vi "AOL Properties parser.vi"(0 "AOL Properties":T4={"AOD 1 thickness (mm)"=118.0, "AOD 2 thickness (mm)"=115.0, "AOD 3 thickness (mm)"=110.0, "AOD 4 thickness (mm)"=135.0, "AOD 1-2 separation (mm)"=135.0, "AOD 2-3 separation (mm)"=135.0, "AOD 3-4 separation (mm)"=15.0, "AOL aperture (mm)"=15.0, "AOL centre wavelength (nm)"=15.0, "AOL centre frequency (MHz)"=15.0, "skewZX"=15.0, "skewZY"=15.0, "magZX"=50.0, "magZY"=50.0, "Diffraction mode"=50.0, "Crystal length (mm)"=15.0, "Acoustic velocity (m/s)"=1.0, "Pair deflection ratio"=1.0, "AOD fill time (us)"=1.0}) -> (14 "Keys setup.DBL":T2=[{"key"="Control FPGA.Clock Freq (MHz)", "Save?"=TRUE, "Default"=240.0}, {"key"="DAQ FPGA.Clock Freq (MHz)", "Save?"=TRUE, "Default"=240.0}], 15 "Values.DBL":dbl[](array[numeric]), 16 "Keys setup.String":T3=[{"key"="Control FPGA.MAC address", "Save?"=TRUE, "Default"="AABBCCDDEEFF"}, {"key"="DAQ FPGA.Target", "Save?"=TRUE, "Default"="RIO0"}, {"key"="XY Stage.COM port", "Save?"=TRUE, "Default"="COM7"}, {"key"="DAQmx Chan.Pockels Control", "Save?"=TRUE, "Default"=""}, {"key"="DAQmx Chan.Hard Shutter", "Save?"=TRUE, "Default"=""}, {"key"="DAQmx Chan.PMT 1", "Save?"=TRUE, "Default"=""}, {"key"="DAQmx Chan.PMT 2", "Save?"=TRUE, "Default"=""}, {"key"="DAQmx Chan.Encoder Trigger", "Save?"=TRUE, "Default"=""}, {"key"="DAQmx Chan.Optional Trigger 1", "Save?"=TRUE, "Default"=""}, {"key"="DAQmx Chan.Optional Trigger 2", "Save?"=TRUE, "Default"=""}, {"key"="DAQmx Chan.Optional Trigger 3", "Save?"=TRUE, "Default"=""}], 17 "Values.Strings":string[](array[string]), 18 "Keys setup.Boolean":T1, 19 "Values.Boolean":bool[](array[boolean]))   [LabVIEW 2013]
uses:
  Typedefs/AOL Properties Cluster.ctl
  Typedefs/Ini file interface (String).ctl
  Typedefs/Ini file interface (DBL).ctl
  Typedefs/Ini file interface (Boolean).ctl
panel:
  # "NOTES:\n1. \"Control FPGA.Ethernet port\" is detected automatically. It is not saved/loaded from file.\n2. \"Control FPGA.Ethernet Opened\" is detected automatically. It is not saved/loaded from file."
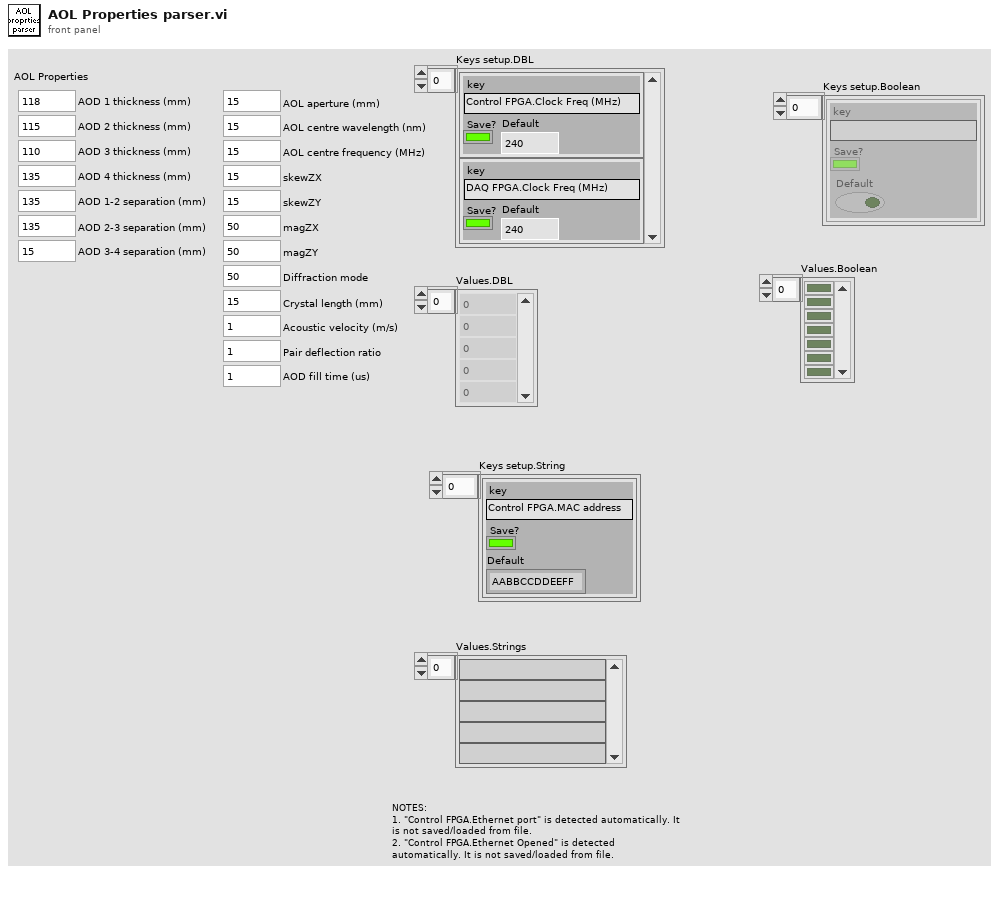
[diagram p1: front panel]
types:
  T1 = typedef "Ini file interface (Boolean).ctl" = cluster{"key":string, "Save?":bool, "Default":bool}[]
  T2 = typedef "Ini file interface (DBL).ctl" = cluster{"key":string, "Save?":bool, "Default":dbl}[]
  T3 = typedef "Ini file interface (String).ctl" = cluster{"key":string, "Save?":bool, "Default":string}[]
  T4 = typedef "AOL Properties Cluster.ctl" = cluster{"AOD 1 thickness (mm)":dbl, "AOD 2 thickness (mm)":dbl, "AOD 3 thickness (mm)":dbl, "AOD 4 thickness (mm)":dbl, "AOD 1-2 separation (mm)":dbl, "AOD 2-3 separation (mm)":dbl, "AOD 3-4 separation (mm)":dbl, "AOL aperture (mm)":dbl, "AOL centre wavelength (nm)":dbl, "AOL centre frequency (MHz)":dbl, "skewZX":dbl, "skewZY":dbl, "magZX":dbl, "magZY":dbl, "Diffraction mode":dbl, "Crystal length (mm)":dbl, "Acoustic velocity (m/s)":dbl, "Pair deflection ratio":dbl, "AOD fill time (us)":dbl}
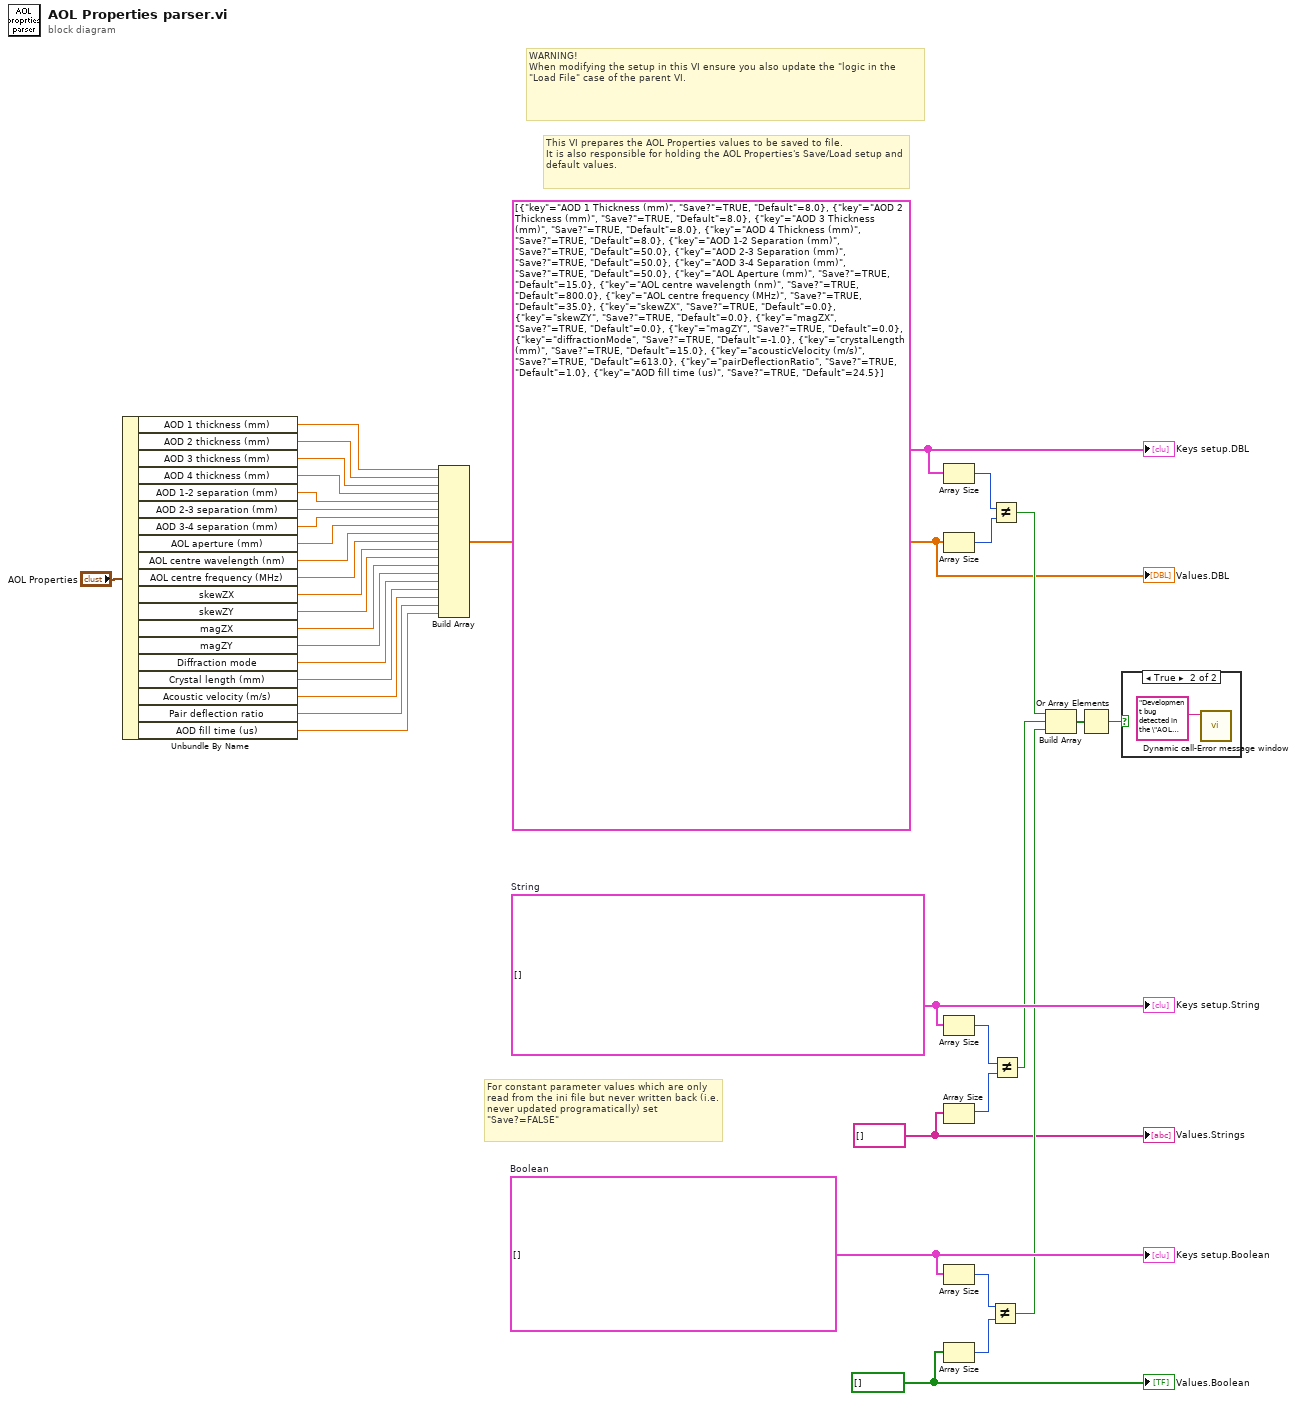
[diagram p0: block diagram]
diagram:
  w2 = T2 [{"key"="AOD 1 Thickness (mm)", "Save?"=TRUE, "Default"=8.0}, {"key"="AOD 2 Thickness (mm)", "Save?"=TRUE, "Default"=8.0}, {"key"="AOD 3 Thickness (mm)", "Save?"=TRUE, "Default"=8.0}, {"key"="AOD 4 Thickness (mm)", "Save?"=TRUE, "Default"=8.0}, {"key"="AOD 1-2 Separation (mm)", "Save?"=TRUE, "Default"=50.0}, {"key"="AOD 2-3 Separation (mm)", "Save?"=TRUE, "Default"=50.0}, {"key"="AOD 3-4 Separation (mm)", "Save?"=TRUE, "Default"=50.0}, {"key"="AOL Aperture (mm)", "Save?"=TRUE, "Default"=15.0}, {"key"="AOL centre wavelength (nm)", "Save?"=TRUE, "Default"=800.0}, {"key"="AOL centre frequency (MHz)", "Save?"=TRUE, "Default"=35.0}, {"key"="skewZX", "Save?"=TRUE, "Default"=0.0}, {"key"="skewZY", "Save?"=TRUE, "Default"=0.0}, {"key"="magZX", "Save?"=TRUE, "Default"=0.0}, {"key"="magZY", "Save?"=TRUE, "Default"=0.0}, {"key"="diffractionMode", "Save?"=TRUE, "Default"=-1.0}, {"key"="crystalLength (mm)", "Save?"=TRUE, "Default"=15.0}, {"key"="acousticVelocity (m/s)", "Save?"=TRUE, "Default"=613.0}, {"key"="pairDeflectionRatio", "Save?"=TRUE, "Default"=1.0}, {"key"="AOD fill time (us)", "Save?"=TRUE, "Default"=24.5}] ("DBL 3")
  w22 = bool[] [] ("appended array")
  w23 = string[] [] ("appended array")
  w36 = T1 []  # Boolean
  w37 = T3 []  # String
  # "WARNING!\nWhen modifying the setup in this VI ensure you also update the \"logic in the \"Load File\" case of the parent VI."
  # "For constant parameter values which are only read from the ini file but never written back (i.e. never updated programatically) set \"Save?=FALSE\""
  # "This VI prepares the AOL Properties values to be saved to file.\nIt is also responsible for holding the AOL Properties's Save/Load setup and default values."
  n1 = Unbundle By Name("AOL Properties") -> ("AOD 1 thickness (mm)"=w21:dbl, "AOD 2 thickness (mm)"=w19:dbl, "AOD 3 thickness (mm)"=w18:dbl, "AOD 4 thickness (mm)"=w17:dbl, "AOD 1-2 separation (mm)"=w16:dbl, "AOD 2-3 separation (mm)"=w15:dbl, "AOD 3-4 separation (mm)"=w14:dbl, "AOL aperture (mm)"=w13:dbl, "AOL centre wavelength (nm)"=w12:dbl, "AOL centre frequency (MHz)"=w11:dbl, "skewZX"=w10:dbl, "skewZY"=w9:dbl, "magZX"=w8:dbl, "magZY"=w7:dbl, "Diffraction mode"=w6:dbl, "Crystal length (mm)"=w5:dbl, "Acoustic velocity (m/s)"=w4:dbl, "Pair deflection ratio"=w3:dbl, "AOD fill time (us)"=w1:dbl)
  n2 = Build Array(w21, w19, w18, w17, w16, w15, w14, w13, w12, w11, w10, w9, w8, w7, w6, w5, w4, w3, w1) -> (w20:dbl[])
  "Values.DBL" <- w20
  n3 = Array Size(array=w2) -> (size(s)=w33:i32)
  n4 = Array Size(array=w20) -> (size(s)=w32:i32)
  n5 = Array Size(array=w37) -> (size(s)=w35:i32)
  n6 = Array Size(array=w23) -> (size(s)=w34:i32)
  n7 = Array Size(array=w36) -> (size(s)=w31:i32)
  n8 = Array Size(array=w22) -> (size(s)=w30:i32)
  n9 = Not Equal?(x=w31, y=w30) -> (x != y?=w28:bool)
  n10 = Not Equal?(x=w33, y=w32) -> (x != y?=w26:bool)
  n11 = Not Equal?(x=w35, y=w34) -> (x != y?=w25:bool)
  n12 = Build Array(w26, w25, w28) -> (w29:bool[])
  n13 = Or Array Elements(Boolean array=w29) -> (logical OR=w27:bool)
  n14 = case shown="True" w27 {
    frame False {
    }
    frame True {
      n15 = call "Dynamic call-Error message window.vi"("Error Message"="Development bug detected in the \"AOL properties parser.vi\".\nPlease correct the set up in this VI.") -> ()  [unwired: 10 in, 1 out]
    }
  }
  "Keys setup.String" <- w37
  "Keys setup.DBL" <- w2
  "Values.Strings" <- w23
  "Keys setup.Boolean" <- w36
  "Values.Boolean" <- w22
